vi "LNLS Control BPM Data.vi"(8 "error in (no error)":errorcluster, 10 "BPM Status (On correction?)":bool[](array[boolean]), 11 "BPM Readings":dbl[](array[numeric])) -> (0 "error out":errorcluster, 3 "BPM Readings Data":T1[](array[typedef]) {"status" format="%08b"})   [LabVIEW 2011, in "LNLS Control VIs.lvlib"]
uses:
  Types Definitions/Type BPM Pre Encode.ctl
  LNLS Control VIs.lvlib
  Type Definitions.lvlib
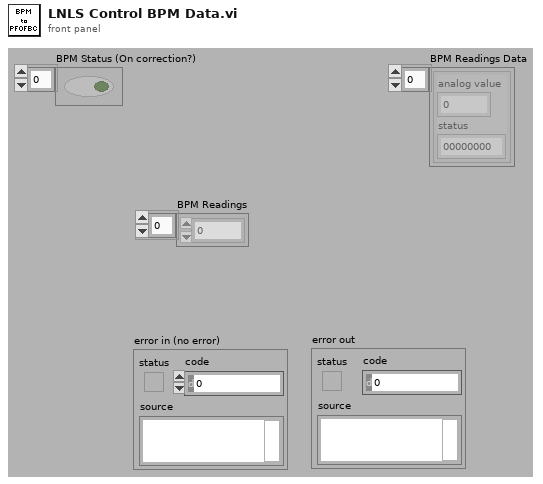
[diagram p1: front panel]
types:
  T1 = typedef "Type Definitions.lvlib/Type BPM Pre Encode.ctl" = cluster{"analog value":dbl, "status":u8}
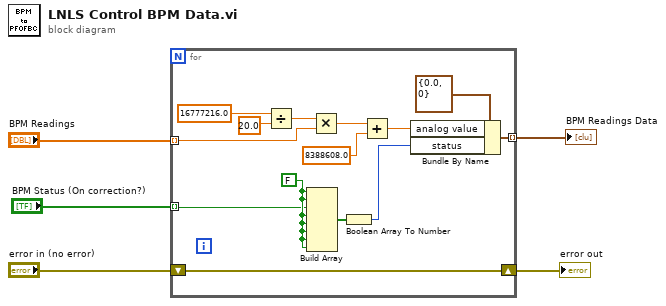
[diagram p0: block diagram]
diagram:
  n1 = for {
    tunnel: [w19] -> w2 mode=indexing
    shift-right: [w17] -> w4
    shift-left: "error in (no error)" -> [w17]
    tunnel: "BPM Readings" -> [w15] mode=indexing
    tunnel: "BPM Status (On correction?)" -> [w7] mode=indexing
    w8 = FALSE ("element")
    n2 = Divide(x=16777216.0, y=20.0) -> (x/y=w10:dbl)
    n3 = Build Array(w8, w8, w7, w8, w8, w8, w8, w8) -> (w9:bool[])
    n4 = Multiply(x=w10, y=w15) -> (x*y=w12:dbl)
    n5 = Boolean Array To Number(Boolean array=w9) -> (number=w6:u32)
    n6 = Add(x=w12, y=8388608.0) -> (x+y=w18:dbl)
    n7 = Bundle By Name(cluster=T1 {"analog value"=0.0, "status"=0} ("LOCON_BIPOLAR_16BITS"), "analog value"=w18, "status"=w6) -> (w19:T1)
  }
  "error out" <- w4
  "BPM Readings Data" <- w2
